vi "DFT.vi"() -> ()   [LabVIEW 2022 SP3]
uses:
  <vilib>/Analysis/baseanly.llb/Complex A x Vector.vi
  <vilib>/Analysis/NI_AALBase.lvlib
panel:
  out "Matrix W":cdb[][](array[numeric])
  out "Output Matrix C":cdb[](array[numeric]) format="%.2f"
  out "Omega":cdb
  out "N":i32
  in  "Input Matrix B":dbl[](array[numeric])
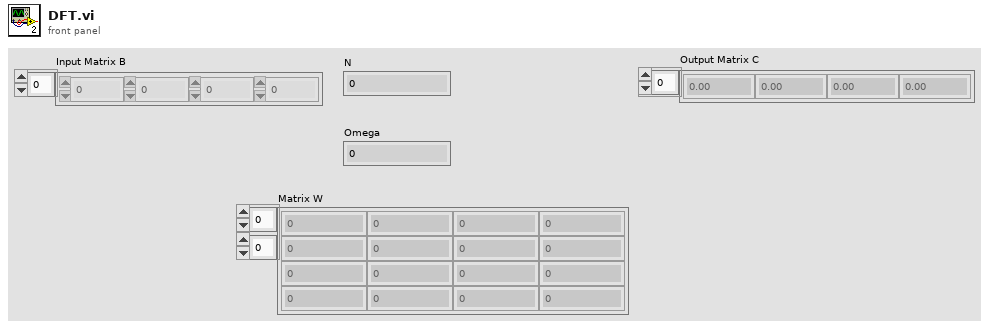
[diagram p1: front panel]
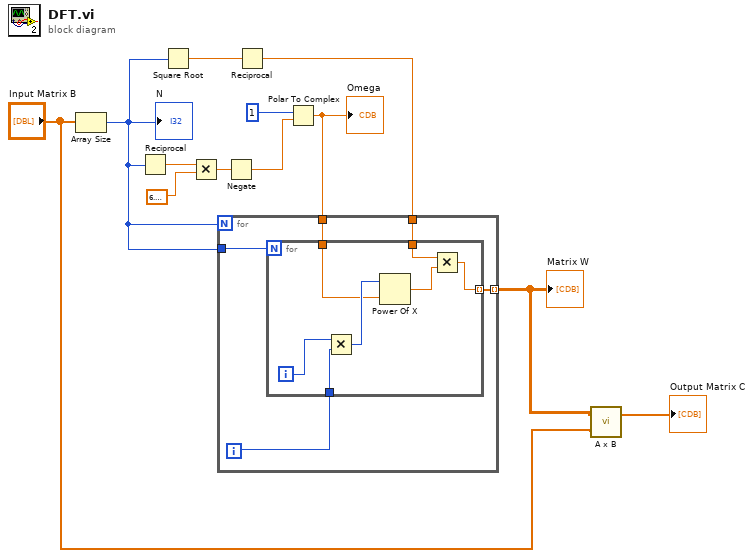
[diagram p0: block diagram]
diagram:
  n1 = Array Size(array="Input Matrix B") -> (size(s)=w3:i32)
  "N" <- w3
  n2 = Reciprocal(x=w3) -> (1/x=w12:dbl)
  n3 = Square Root(x=w3) -> (sqrt(x)=w2:dbl)
  n4 = Multiply(x=w12, y=6.283185307179586) -> (x*y=w9:dbl)
  n5 = Negate(x=w9) -> (-x=w8:dbl)
  n6 = Reciprocal(x=w2) -> (1/x=w1:dbl)
  n7 = Polar To Complex(1:w8, 2:1) -> (0:w7:cdb)
  "Omega" <- w7
  n8 = for {
    N: w3 -> [_]
    tunnel: w3 -> [w17]
    tunnel: w7 -> [w15]
    tunnel: [w14] -> w4 mode=indexing
    tunnel: w1 -> [w13]
    i -> [w16]
    n9 = for {
      N: w17 -> [_]
      tunnel: w16 -> [w24]
      tunnel: w15 -> [w21]
      tunnel: [w18] -> w14 mode=indexing
      tunnel: w13 -> [w20]
      i -> [w23]
      n10 = Multiply(x=w23, y=w24) -> (x*y=w22:i32)
      n11 = Power Of X(1:w21, 2:w22) -> (0:w19:cdb)
      n12 = Multiply(x=w20, y=w19) -> (x*y=w18:cdb)
    }
  }
  "Matrix W" <- w4
  n13 = call-poly <vilib>:"A x B.vi"("Vector"="Input Matrix B", "A"=w4) -> ("A x Vector"=→"Output Matrix C":cdb[])  [unwired: 1 out]
